vi "Read Local Resource.vi"(8 "error in (no error)":errorcluster, 11 "4081 in":refnum<class "4081.lvclass">) -> (0 "error out":errorcluster, 2 "Local Resource":refnum<k15>, 3 "4081 out":refnum<class "4081.lvclass">)   [LabVIEW 2019, in "4081.lvlib" / "4081.lvclass"]
uses:
  Library/4081.lvclass
  Library/4081.lvclass/4081.ctl
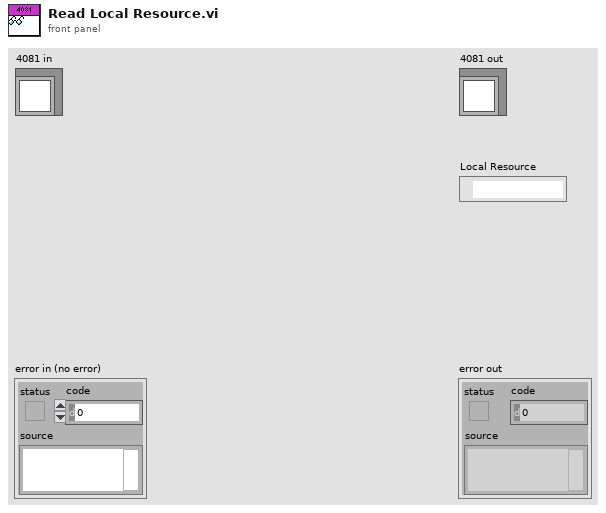
[diagram p1: front panel]
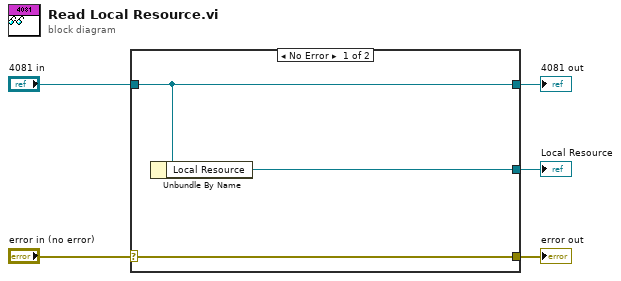
[diagram p0: block diagram]
diagram:
  n1 = case shown="No Error" "error in (no error)" {
    selector: "error in (no error)" -> [w8 w9]
    tunnel: [w8 w9] -> w4
    tunnel: [w7 w10] -> w2
    tunnel: "4081 in" -> [w7 w10]
    tunnel: [w6 _] -> w1
    frame No Error {
      n2 = Unbundle By Name(w7) -> ("Local Resource"=w6:refnum<k15>)
    }
    frame Error {
    }
  }
  "error out" <- w4
  "4081 out" <- w2
  "Local Resource" <- w1
